vi "GT_SetVel.vi"(3 "vel":dbl, 4 "axis in":T1=1 items=["Axis Control"=0, "Axis 1"=1, "Axis 2"=2, "Axis 3"=3, "Axis 4"=4, "Axis 5"=5, "Axis 6"=6, "Axis 7"=7, "Axis 8"=8, "Vector Space Control"=16, "Vector Space 1"=17, "Vector Space 2"=18, "Vector Space 3"=19, "Vector Space 4"=20], 5 "rtn_In":cluster{"rtn":i16, "Func":string}) -> (1 "axis out":T1=1 items=["Axis Control"=0, "Axis 1"=1, "Axis 2"=2, "Axis 3"=3, "Axis 4"=4, "Axis 5"=5, "Axis 6"=6, "Axis 7"=7, "Axis 8"=8, "Vector Space Control"=16, "Vector Space 1"=17, "Vector Space 2"=18, "Vector Space 3"=19, "Vector Space 4"=20], 2 "rtn_Out":cluster{"rtn":i16, "Func":string})   [LabVIEW 2014]
uses:
  <vilib>/Motion/FlexMotion/CustomControls/CustomControls.llb/AxisOrVectorSpaceControl To Control.flx
  VC6/gts.dll
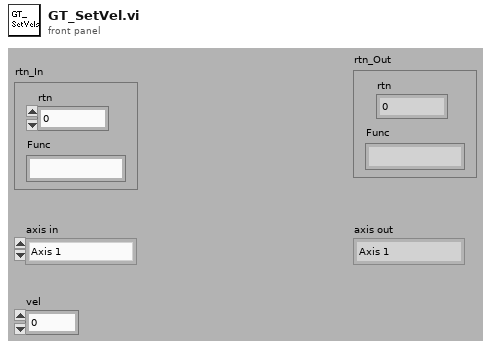
[diagram p1: front panel]
types:
  T1 = typedef "AxisOrVectorSpaceControl To Control.flx" = u16
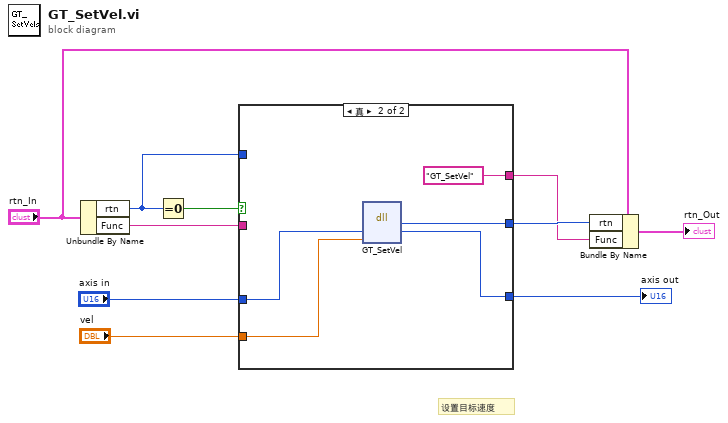
[diagram p0: block diagram]
diagram:
  # "设置目标速度"
  n1 = Unbundle By Name("rtn_In") -> ("rtn"=w1:i16, "Func"=w9:string)
  n2 = Equal To 0?(x=w1) -> (x = 0?=w10:bool)
  n3 = case shown="真" w10 {
    tunnel: w9 -> [w13 _]
    tunnel: [w12 w18] -> w6
    tunnel: "axis in" -> [w11 w17]
    tunnel: "vel" -> [_ w16]
    tunnel: [w11 w15] -> w3
    tunnel: [w13 "GT_SetVel" ("Func")] -> w2
    tunnel: w1 -> [w12 _]
    frame False {
    }
    frame True {
      n4 = dll-call lib="PTH2Fabs DNewGTS AC-800LWin7版源程序-20170926gts85VC6gts.dll" fn="GT_SetVel"("profile"=w17, "vel"=w16) -> ("rtn"=w18:i16, "profile"=w15:i16)  [unwired: 4 in, 2 out]
    }
  }
  "axis out" <- w3
  n5 = Bundle By Name(cluster="rtn_In", "rtn"=w6, "Func"=w2) -> (→"rtn_Out":cluster{"rtn":i16, "Func":string})
